vi "mupExpr sglExpr multiVar bulkMode.vi"() -> ()   [LabVIEW 2015]
uses:
  mupExpr/mupExpr.lvclass
  mupExpr/mupExpr.lvclass/mupExpr.ctl
  mupExpr/Eval_MultiVar_BulkMode.vi
  mupExpr/SetVarVal_Array.vi
  mupLib/mupEvalBulk.vi
  mupLib/mupSetVarValue_Array.vi
  mupLib/mupCheckError.vi
  <vilib>/Utility/error.llb/Error Cluster From Error Code.vi
panel:
  out "error out":errorcluster
  out "Results":dbl[](array[numeric]) format="%#_13g"
  out "Variable Names":string[](array[string])
  in  "Expression":string="a*x+b"
  in  "Variable Values":dbl[][](array[numeric])=[[1.0, 1.0, 1.0, 1.0], [1.0, 2.0, 3.0, 4.0], [5.0, 5.0, 5.0, 5.0]] format="%#_13g"
  # "(one row per variable)"
  # "This example demonstrates bulk-mode evaluation of a multi-variable expression.\n\n- Enter an expression composed of any number of variables\n- Enter the set of values for each variable (variables are listed in alphabetical order)\n- Hit run to evaluate the expression"
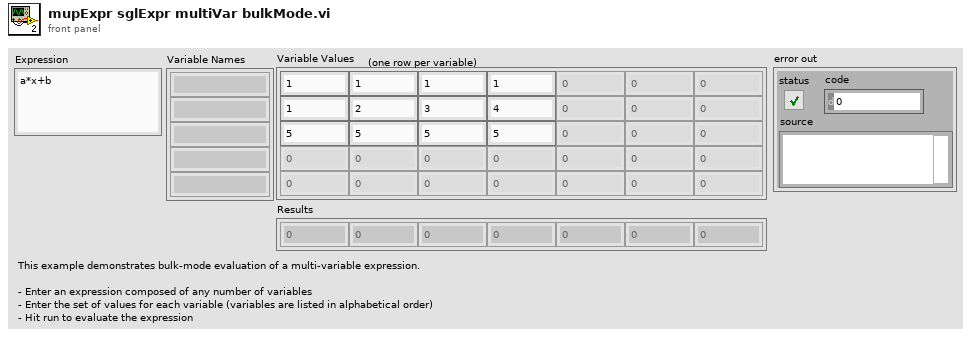
[diagram p1: front panel]
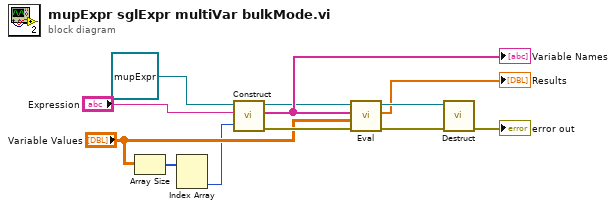
[diagram p0: block diagram]
diagram:
  n1 = Array Size(array="Variable Values") -> (size(s)=w3:i32[])
  n2 = Index Array(array=w3) -> (element #2=w2:i32)  [unwired: 2 in, 1 out]
  n3 = call-dynamic "Construct.vi"("Bulk Size (1)"=w2, "Expression"="Expression", "muExpr in"=refnum<class "mupExpr.lvclass"> refnum) -> ("error out"=w8:errorcluster, "Variable Names"=w9:string[], "mupExpr out"=w7:refnum<class "mupExpr.lvclass">)  [unwired: 5 in, 1 out]
  "Variable Names" <- w9
  n4 = call-poly "Eval.vi"("error in (no error)"=w8, "varValues"="Variable Values", "varNames"=w9, "muExpr in"=w7) -> ("error out"=w10:errorcluster, "Result"=→"Results":dbl[], "muExpr out"=w11:refnum<class "mupExpr.lvclass">)  [unwired: 5 in]
  n5 = call-dynamic "Destruct.vi"("error in (no error)"=w10, "muExpr in"=w11) -> ("error out"=→"error out":errorcluster)  [unwired: 9 in]
